vi "VI Tree - error__ogtk.vi"   [LabVIEW 2012]
uses:
  <userlib>/_OpenG.lib/error/error.llb/Filter Error Codes (Array)__ogtk.vi
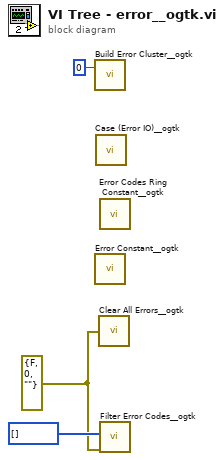
[diagram p0: block diagram]
diagram:
  w1 = errorcluster {"status"=FALSE, "code"=0, "source"=""} ("error in")
  n1 = call <userlib>:"Build Error Cluster__ogtk.vi"("code"=0) -> ()  [unwired: 1 in, 1 out]
  n2 = call <userlib>:"Error Constant__ogtk.vi"() -> ()  [unwired: 1 in]
  n3 = call <userlib>:"Case (Error IO)__ogtk.vi"() -> ()  [unwired: 1 in]
  n4 = call <userlib>:"Clear All Errors__ogtk.vi"("Error In"=w1) -> ()  [unwired: 3 in, 1 out]
  n5 = call <userlib>:"Error Codes Ring Constant__ogtk.vi"() -> ()  [unwired: 1 in]
  n6 = call-poly <userlib>:"Filter Error Codes__ogtk.vi"("Error In"=w1, "Error Codes to Filter"=i32[] [] ("error codes to filter")) -> ()  [unwired: 7 in, 3 out]
